vi "Generate Blend Points.vi"(6 "Index":i32, 8 "Speeds":T2={"maxV (fps)"=20.0, "Accel Limit (fps^2)"=20.0, "Initial V (fps)"=0.0, "Sample Period (s)"=0.02, "Jerk Limit (fps^3)"=0.0, "Jerk Distances"={"distance (ft)"=0.0, 0.0, 0.0}, "Jerk Distances"={"distance (ft)"=0.0, 0.0, 0.0}}, 9 "Initial Point":cluster{"x":dbl, "y":dbl, "th":dbl}={"x"=1.0, "y"=2.0, "th"=30.0}, 11 "Blend Info":T1) -> (0 "Speeds Out":T2={"maxV (fps)"=20.0, "Accel Limit (fps^2)"=20.0, "Initial V (fps)"=0.0, "Sample Period (s)"=0.02, "Jerk Limit (fps^3)"=0.0, "Jerk Distances"={"distance (ft)"=0.0, 0.0, 0.0}, "Jerk Distances"={"distance (ft)"=0.0, 0.0, 0.0}}, 3 "Trajectory Segment":T3)   [LabVIEW 2018]
uses:
  BlendType.ctl
panel:
  out "XY Graph":cluster{cluster{dbl, dbl}[]}[](graph)
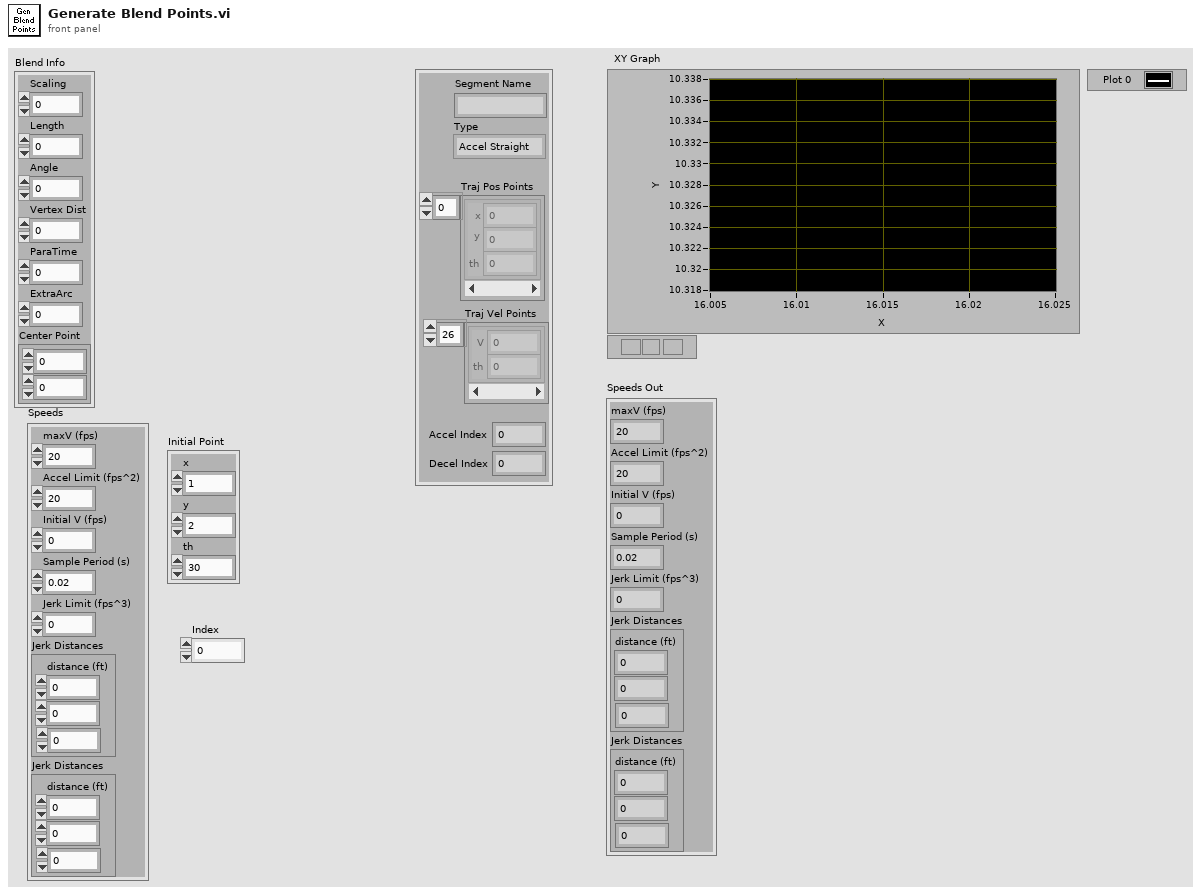
[diagram p1: front panel]
types:
  T1 = typedef "BlendType.ctl" = cluster{"Scaling":dbl, "Length":dbl, "Angle":dbl, "Vertex Dist":dbl, "ParaTime":dbl, "ExtraArc":dbl, "Center Point":cluster{dbl, dbl}}
  T2 = cluster{"maxV (fps)":dbl, "Accel Limit (fps^2)":dbl, "Initial V (fps)":dbl, "Sample Period (s)":dbl, "Jerk Limit (fps^3)":dbl, "Jerk Distances":cluster{"distance (ft)":dbl, dbl, dbl}, "Jerk Distances":cluster{"distance (ft)":dbl, dbl, dbl}}
  T3 = cluster{"Segment Name":string, "Type":enum16{"Accel Straight", "Const Straight", "Blend", "Circle"}, "Traj Pos Points":cluster{"x":dbl, "y":dbl, "th":dbl}[], "Traj Vel Points":cluster{"V":dbl, "th":dbl}[], "Accel Index":i32, "Decel Index":i32}
  T4 = enum16{"Accel Straight", "Const Straight", "Blend", "Circle"}
  T5 = cluster{string, "Type":enum16{"Accel Straight", "Const Straight", "Blend", "Circle"}, cluster{dbl, dbl, dbl}[], cluster{dbl, dbl}[], "Accel Index":i32, "Decel Index":i32}
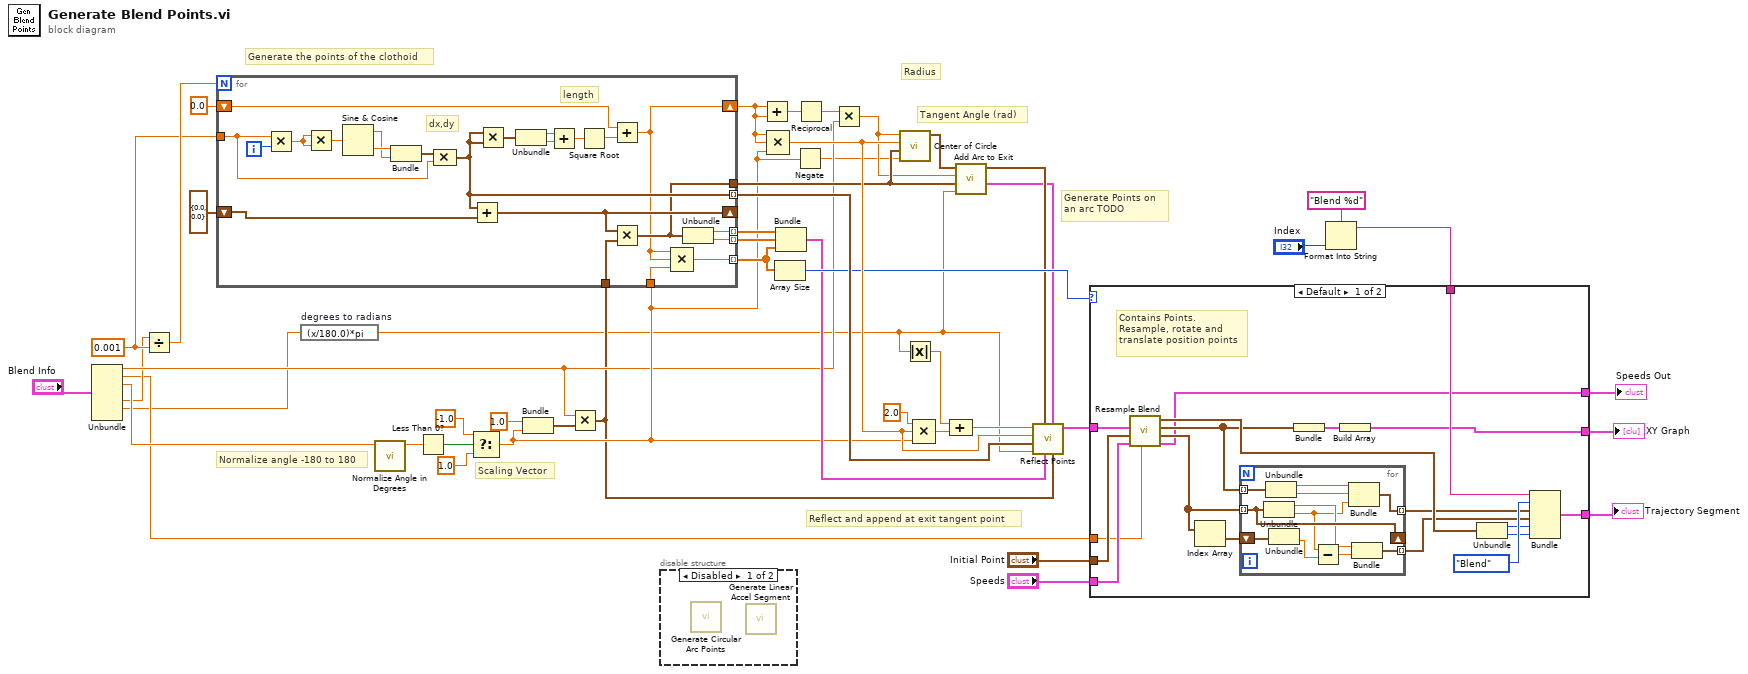
[diagram p0: block diagram]
diagram:
  w15 = 0.001
  # "Generate Points on \nan arc TODO"
  # "Reflect and append at exit tangent point"
  # "Scaling Vector"
  # "Normalize angle -180 to 180"
  # "Radius"
  # "Tangent Angle (rad)"
  # "Generate the points of the clothoid"
  n1 = Unbundle("Blend Info") -> ("Scaling"=w13:dbl, "Length"=w10:dbl, "Angle"=w12:dbl, "ParaTime"=w11:dbl, "ExtraArc"=w5:dbl)  [unwired: 2 out]
  n2 = Divide(x=w11, y=w15) -> (x/y=w47:dbl)
  n3 = expression code="(x/180.0)*pi" "degrees to radians"(w5) -> (w1:dbl)
  n4 = call "Normalize Angle in Degrees.vi"("Angle deg"=w12) -> ("Angle"=w26:dbl)  [unwired: 10 in]
  n5 = Less Than 0?(x=w26) -> (x < 0?=w29:bool)
  n6 = Select(t=-1.0, s=w29, f=1.0) -> (s? t:f=w20:dbl)
  n7 = Bundle(1.0, w20) -> (w27:cluster{dbl, dbl})  [unwired: 1 in]
  n8 = Multiply(x=w13, y=w27) -> (x*y=w3:cluster{dbl, dbl})
  n9 = for {
    N: w47 -> [_]
    shift-right: [w64] -> _
    shift-left: cluster{dbl, dbl} {0.0, 0.0} -> [w66]
    tunnel: w15 -> [w63]
    shift-right: [w53] -> w45
    shift-left: 0.0 -> [w58]
    tunnel: [w54] -> w40
    tunnel: [w56] -> w46 mode=indexing
    tunnel: w3 -> [w55]
    tunnel: [w50] -> w24 mode=indexing
    tunnel: [w49] -> w25 mode=indexing
    tunnel: w20 -> [w52]
    tunnel: [w51] -> w22 mode=indexing
    i -> [w71]
    # "length"
    # "dx,dy"
    n10 = Multiply(x=w63, y=w71) -> (x*y=w65:dbl)
    n11 = Multiply(x=w65, y=w65) -> (x*y=w70:dbl)
    n12 = Sine & Cosine(0:w70) -> (1:w68:dbl, 2:w69:dbl)
    n13 = Bundle(w69, w68) -> (w67:cluster{dbl, dbl})  [unwired: 1 in]
    n14 = Compound Arithmetic op=MULTIPLY(w67, w63) -> (w56:cluster{dbl, dbl})
    n15 = Add(x=w56, y=w66) -> (x+y=w64:cluster{dbl, dbl})
    n16 = Multiply(x=w56, y=w56) -> (x*y=w62:cluster{dbl, dbl})
    n17 = Unbundle(w62) -> (w61:dbl, w60:dbl)
    n18 = Add(x=w61, y=w60) -> (x+y=w59:dbl)
    n19 = Square Root(x=w59) -> (sqrt(x)=w57:dbl)
    n20 = Add(x=w58, y=w57) -> (x+y=w53:dbl)
    n21 = Multiply(x=w64, y=w55) -> (x*y=w54:cluster{dbl, dbl})
    n22 = Compound Arithmetic op=MULTIPLY(w53, w53, w52) -> (w51:dbl)
    n23 = Unbundle(w54) -> (w50:dbl, w49:dbl)
  }
  n24 = disable-structure shown="Disabled" {
    frame Disabled {
      n25 = call "Generate Circular Arc Points.vi"() -> ()  [unwired: 9 in, 3 out]
      n26 = call "Generate Linear Accel Segment.vi"() -> ()  [unwired: 8 in, 4 out]
    }
    frame Enabled {
    }
  }
  n27 = Add(x=w45, y=w45) -> (x+y=w44:dbl)
  n28 = Compound Arithmetic op=MULTIPLY(w45, w45, w20) -> (w42:dbl)
  n29 = Array Size(array=w22) -> (size(s)=w33:i32)
  n30 = Bundle(w24, w25, w22) -> (w23:cluster{dbl[], dbl[], dbl[]})  [unwired: 1 in]
  n31 = Negate(x=w20) -> (-x=w6:dbl)
  n32 = Reciprocal(x=w44) -> (1/x=w43:dbl)
  n33 = Multiply(x=w43, y=w13) -> (x*y=w39:dbl)
  n34 = call "Center of Circle.vi"("Sign"=w6, "Tangent Point"=w40, "Tangent Angle"=w42, "Radius"=w39) -> ("Center Point"=w41:cluster{dbl, dbl})  [unwired: 7 in]
  n35 = Absolute Value(x=w1) -> (abs(x)=w4:dbl)
  n36 = Compound Arithmetic op=MULTIPLY(2.0, w42, w20) -> (w16:dbl)
  n37 = Compound Arithmetic op=ADD(w4, w16) -> (w17:dbl)
  n38 = call "Add Arc to Exit.vi"("Additional circle arc (rad)"=w1, "Tangent Point"=w40, "Radius"=w39, "Center Point"=w41) -> ("Point Arrays"=w2:cluster{dbl[], dbl[], dbl[]}, "Blend Exit Point"=w19:cluster{dbl, dbl})  [unwired: 6 in]
  n39 = call "Reflect Points.vi"("Scaling Vector"=w3, "Arc Point Arrays"=w2, "Blend Point Arrays"=w23, "Blend Exit Point"=w19, "Extra Arc rad"=w1, "Delta Points"=w46, "Tangent Angle (rad)"=w42, "Angle"=w17) -> ("Point Arrays"=w21:cluster{dbl[], dbl[], dbl[]})  [unwired: 3 in]
  n40 = Format Into String(format string="Blend %d", "Index") -> (resulting string=w9:string)  [unwired: 2 in, 1 out]
  n41 = case shown="Default" w33 {
    tunnel: "Initial Point" -> [w85 _]
    tunnel: [w88 _] -> w36
    tunnel: "Speeds" -> [w83 w101]
    tunnel: w9 -> [w87 _]
    tunnel: [w86 _] -> w34
    tunnel: [w73 w101] -> w32
    tunnel: w21 -> [w72 _]
    tunnel: w10 -> [w82 _]
    frame Default {
      # "Contains Points.\nResample, rotate and\ntranslate position points"
      n42 = call "Resample Blend.vi"("Length"=w82, "Speeds"=w83, "Initial Point"=w85, "Point Arrays"=w72) -> ("Speeds Out"=w73:T2, "Vel Points"=w74:cluster{dbl, dbl}[], "Points"=w75:cluster{dbl, dbl}[], "Indices"=w81:cluster{"Accel Index":i32, "Decel Index":i32})  [unwired: 4 in]
      n43 = Index Array(array=w74) -> (element=w78:cluster{dbl, dbl})  [unwired: 1 in]
      n44 = for {
        tunnel: w75 -> [w100] mode=indexing
        tunnel: [w97] -> w76 mode=indexing
        tunnel: w74 -> [w93] mode=indexing
        shift-right: [w93] -> _
        shift-left: w78 -> [w95]
        tunnel: [w90] -> w77 mode=indexing
        n45 = Unbundle(w93) -> (w92:dbl, w91:dbl)
        n46 = Unbundle(w100) -> (w99:dbl, w98:dbl)
        n47 = Unbundle(w95) -> (w96:dbl)  [unwired: 1 out]
        n48 = Subtract(x=w91, y=w96) -> (x-y=w94:dbl)
        n49 = Bundle(w99, w98, w91) -> (w97:cluster{dbl, dbl, dbl})  [unwired: 1 in]
        n50 = Bundle(w92, w94) -> (w90:cluster{dbl, dbl})  [unwired: 1 in]
      }
      n51 = Bundle("Points"=w75) -> (w89:cluster{"Points":cluster{dbl, dbl}[]})  [unwired: 1 in]
      n52 = Build Array(w89) -> (w86:cluster{"Points":cluster{dbl, dbl}[]}[])
      n53 = Unbundle(w81) -> ("Accel Index"=w80:i32, "Decel Index"=w79:i32)
      n54 = Bundle(w87, "Type"=T4."Blend", w76, w77, "Accel Index"=w80, "Decel Index"=w79) -> (w88:T5)  [unwired: 1 in]
    }
    frame 0 {
    }
  }
  "Trajectory Segment" <- w36
  "XY Graph" <- w34
  "Speeds Out" <- w32
